vi "Camera Control.vi"(1 "Camera Data":T1) -> (0 "Camera Data out":T1)   [LabVIEW 2012]
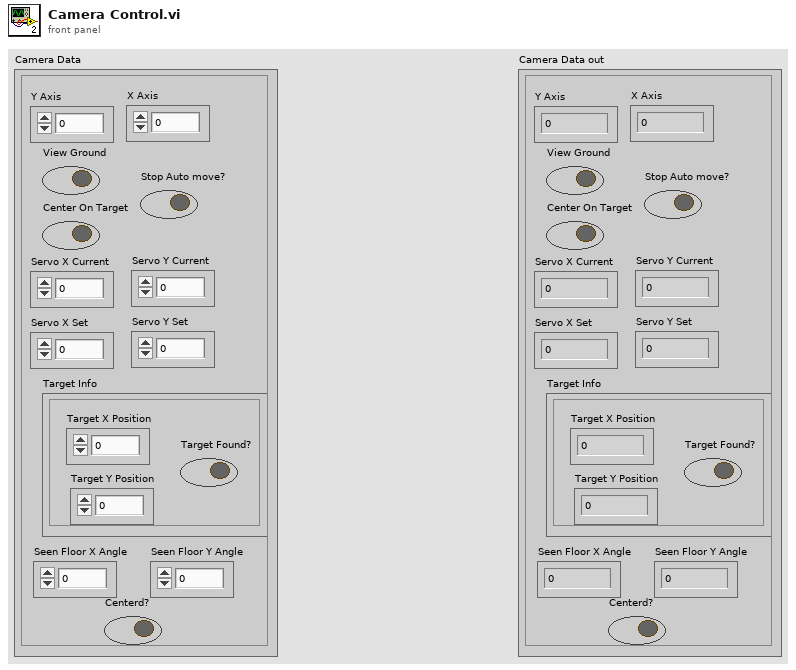
[diagram p1: front panel]
types:
  T1 = cluster{"Y Axis":dbl, "X Axis":dbl, "View Ground":bool, "Center On Target":bool, "Stop Auto move?":bool, "Servo X Current":dbl, "Servo Y Current":dbl, "Target Info":cluster{"Target Found?":bool, "Target X Position":dbl, "Target Y Position":dbl}, "Seen Floor X Angle":dbl, "Seen Floor Y Angle":dbl, "Centerd?":bool, "Servo X Set":dbl, "Servo Y Set":dbl}
  T2 = cluster{"Target Found?":bool, "Target X Position":dbl, "Target Y Position":dbl}
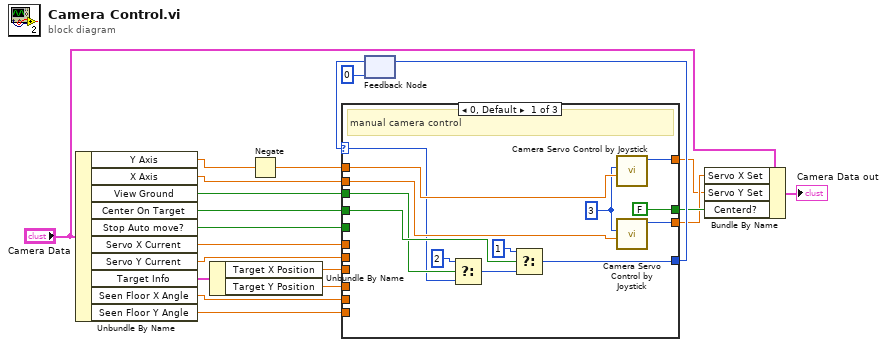
[diagram p0: block diagram]
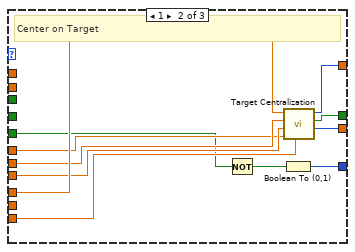
[diagram p2: hidden frame]
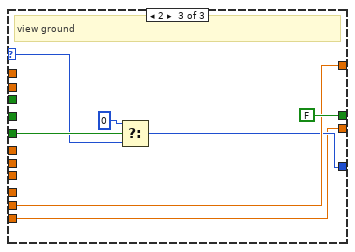
[diagram p3: hidden frame]
diagram:
  n1 = Unbundle By Name("Camera Data") -> ("Y Axis"=w16:dbl, "X Axis"=w15:dbl, "View Ground"=w10:bool, "Center On Target"=w11:bool, "Stop Auto move?"=w14:bool, "Servo X Current"=w6:dbl, "Servo Y Current"=w8:dbl, "Target Info"=w21:T2, "Seen Floor X Angle"=w13:dbl, "Seen Floor Y Angle"=w12:dbl)
  n2 = Unbundle By Name(w21) -> ("Target X Position"=w7:dbl, "Target Y Position"=w9:dbl)
  n3 = Negate(x=w16) -> (-x=w20:dbl)
  n4 = feedback #1(i16 0) -> (w17:i16)
  n5 = case shown="0, Default" w17 {
    selector: w17 -> [w22 _ w48]
    tunnel: w12 -> [_ w41 w46]
    tunnel: w13 -> [_ _ w51]
    tunnel: [w23 w40 w51] -> w1
    tunnel: w20 -> [w25 _ _]
    tunnel: w8 -> [_ w44 _]
    tunnel: w15 -> [w34 _ _]
    tunnel: w6 -> [_ w42 _]
    tunnel: w9 -> [_ w45 _]
    tunnel: w7 -> [_ w43 _]
    tunnel: [FALSE ("centered") w37 FALSE ("centered")] -> w3
    tunnel: [w27 w38 w47] -> w19
    tunnel: w14 -> [_ w36 w50]
    tunnel: w11 -> [w29 _ _]
    tunnel: w10 -> [w28 _ _]
    tunnel: [w26 w35 w46] -> w2
    frame 0, Default {
      w24 = 3 ("y")
      # "manual camera control"
      n6 = Select(t=i16 2, s=w28, f=w22) -> (s? t:f=w32:i16)
      n7 = Select(t=i16 1, s=w29, f=w32) -> (s? t:f=w27:i16)
      n8 = call "Camera Servo Control by Joystick.vi"("axis control"=w25, "max jump angle"=w24) -> ("angle set"=w23:i32)  [unwired: 9 in]
      n9 = call "Camera Servo Control by Joystick.vi"("axis control"=w34, "max jump angle"=w24) -> ("angle set"=w26:i32)  [unwired: 9 in]
    }
    frame 1 {
      # "Center on Target"
      n10 = Not(x=w36) -> (.not. x?=w39:bool)
      n11 = Boolean To (0,1)(Boolean=w39) -> (0, 1=w38:i16)
      n12 = call "Target Centralization.vi"("X axis center angle"=w41, "Servo Get Angle X"=w42, "Target Position X"=w43, "Servo Get Angle Y"=w44, "Target Position Y"=w45) -> ("Servo Angle Set Point X"=w35:i32, "centered"=w37:bool, "Servo Angle Set Point Y"=w40:i32)  [unwired: 1 in, 2 out]
    }
    frame 2 {
      # "view ground"
      n13 = Select(t=i16 0, s=w50, f=w48) -> (s? t:f=w47:i16)
    }
  }
  n14 = feedback-in #1(w19) -> ()
  n15 = Bundle By Name(cluster="Camera Data", "Servo X Set"=w2, "Servo Y Set"=w1, "Centerd?"=w3) -> (→"Camera Data out":T1)
